vi "Read Parent Attributes.vi"(11 "Actor in":refnum<class "Actor.lvclass">) -> (2 "Parent Attributes":refnum<class "Attributes.lvclass">)   [LabVIEW 2025, in "jettl.lvlib" / "Actor.lvlib" / "Actor.lvclass"]
uses:
  Actor.lvclass
  Attributes/Attributes/Attributes.lvclass
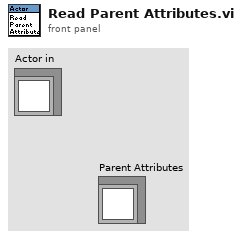
[diagram p1: front panel]
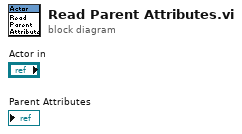
[diagram p0: block diagram]
diagram:
